vi "写入外设配置.vi"(8 "error in (no error)":errorcluster, 10 "外设配置":T1 {"光谱仪类型" items=["1型", "2型"]; "泵阀量" items=["9通"=9, "12通"=12]; "泵类型" items=["1型", "2型"]}, 11 "MB session in":refnum<class "MB_Master.lvclass">) -> (0 "error out":errorcluster, 3 "MB session out":refnum<class "MB_Master.lvclass">)   [LabVIEW 2016, in "斯坦道总磷.lvlib"]
uses:
  <vilib>/Plasmionique/MB Master/MB_Master/MB_Master.lvclass
  <vilib>/Plasmionique/MB Master/MB_Master_Serial/MB_Master_Serial.lvclass
  C:/Program Files (x86)/National Instruments/LabVIEW 2016/vi.lib/Plasmionique/MB Master/MB_Master/MB_Master.lvclass
  <vilib>/Plasmionique/MB Master/MB Master.lvlib
panel:
  in  "VISA Resource":refnum<visa-resource-name>
  in  "引用选择":enum16{"MB引用", "自建引用"}(ring)
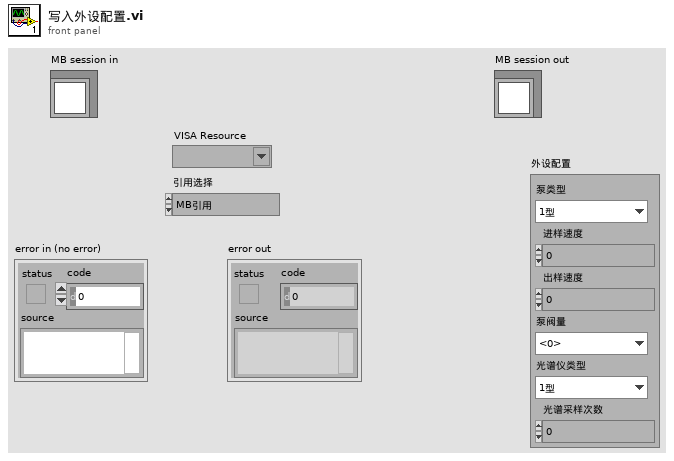
[diagram p1: front panel]
types:
  T1 = cluster{"泵类型":u16, "进样速度":u32, "出样速度":u32, "泵阀量":u16, "光谱仪类型":u16, "光谱采样次数":u8}
  T2 = cluster{"baud rate (bps)":u32, "stop bits":u16, "parity":u16, "flow control":u16, "timeout":u32, "retries":i32}
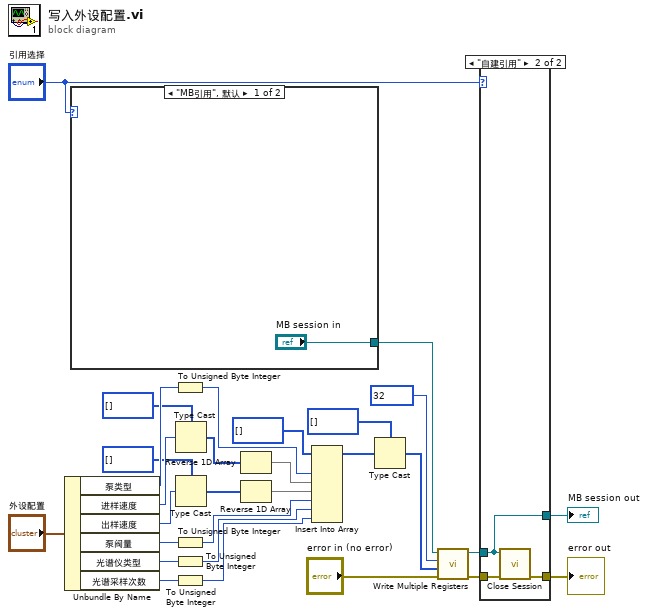
[diagram p0: block diagram]
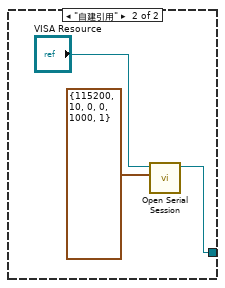
[diagram p3: hidden frame]
diagram:
  n1 = Unbundle By Name("外设配置") -> ("泵类型"=w28:u16, "进样速度"=w27:u32, "出样速度"=w24:u32, "泵阀量"=w17:u16, "光谱仪类型"=w15:u16, "光谱采样次数"=w14:u8)
  n2 = case shown="\"MB引用\", 默认" "引用选择" {
    tunnel: ["MB session in" w33] -> w7
    frame "MB引用", Default {
    }
    frame "自建引用" {
      n3 = call <vilib>:"Open Serial Session.vi"("Serial Config"=T2 {"baud rate (bps)"=115200, "stop bits"=10, "parity"=0, "flow control"=0, "timeout"=1000, "retries"=1}, "VISA Resource"="VISA Resource") -> ("MB_Serial session"=w33:refnum<class "MB_Master_Serial.lvclass">)  [unwired: 8 in, 1 out]
    }
  }
  n4 = To Unsigned Byte Integer(number=w28) -> (unsigned 8bit integer=w21:u8)
  n5 = To Unsigned Byte Integer(number=w17) -> (unsigned 8bit integer=w16:u8)
  n6 = To Unsigned Byte Integer(number=w15) -> (unsigned 8bit integer=w13:u8)
  n7 = To Unsigned Byte Integer(number=w14) -> (unsigned 8bit integer=w12:u8)
  n8 = Type Cast(type=u8[] [], x=w27) -> (*(type *) &x=w23:u8[])
  n9 = Type Cast(type=u8[] [], x=w24) -> (*(type *) &x=w22:u8[])
  n10 = Reverse 1D Array(array=w23) -> (reversed array=w19:u8[])
  n11 = Reverse 1D Array(array=w22) -> (reversed array=w18:u8[])
  n12 = Insert Into Array(array=u8[] [] ("数组"), new element #1=w21, new element #2=w19, new element #3=w18, new element #4=w16, new element #5=w13, new element #6=w12) -> (w11:u8[])  [unwired: 1 in]
  n13 = Type Cast(type=u16[] [], x=w11) -> (*(type *) &x=w1:u16[])
  n14 = call <vilib>:"Write Multiple Registers.vi"("error in (no error)"="error in (no error)", "values"=w1, "starting address"=u16 32, "MB session in"=w7) -> ("error out"=w4:errorcluster, "MB session out"=w6:refnum<class "MB_Master.lvclass">)  [unwired: 6 in]
  n15 = case shown="\"自建引用\"" "引用选择" {
    tunnel: w6 -> [w34 w36]
    tunnel: w4 -> [w35 w38]
    tunnel: [w35 w37] -> w3
    tunnel: [w34 w36] -> w2
    frame "MB引用", Default {
    }
    frame "自建引用" {
      n16 = call-dynamic "Close Session.vi"("error in (no error)"=w38, "MB session in"=w36) -> ("error out"=w37:errorcluster)  [unwired: 9 in]
    }
  }
  "MB session out" <- w2
  "error out" <- w3
